vi "Test Get Audio Device Configuration.vi"(8 "error in (no error)":errorcluster) -> (0 "error out":errorcluster, 3 "Pass?":bool)   [LabVIEW 2020]
uses:
  G-Audio/Controls/Audio Device Config.ctl
  G-Audio/Controls/Audio Device Format.ctl
  G-Audio/Controls/Audio Device Advanced Config.ctl
  G-Audio/Private/Result To Error.vi
  G-Audio/Private/Audio Device Refnum To Value.vi
  <vilib>/Utility/error.llb/Error Cluster From Error Code.vi
  G-Audio/G-Audio.lvlib
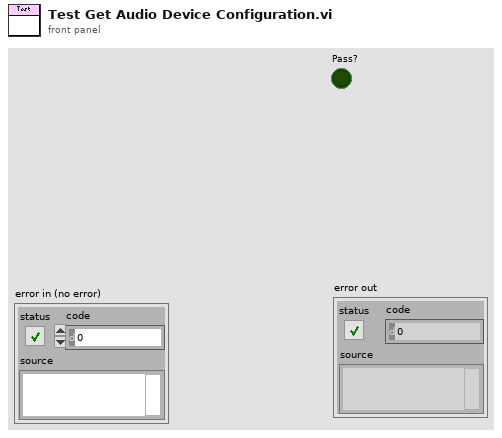
[diagram p1: front panel]
types:
  T1 = typedef "G-Audio.lvlib/Audio Device Advanced Config.ctl" = cluster{"Exclusive Mode":bool, "Period Size":u32, "Num Periods":u32}
  T2 = typedef "G-Audio.lvlib/Audio Device Config.ctl" = cluster{"Sample Rate (Hz)":u32, "Channels":u32, "Format":T3}
  T3 = typedef "G-Audio.lvlib/Audio Device Format.ctl" = enum16{"Native", "U8", "I16", "I32", "SGL"}
  T4 = typedef "G-Audio.lvlib/Audio Device Refnum.ctl" = refnum<file>
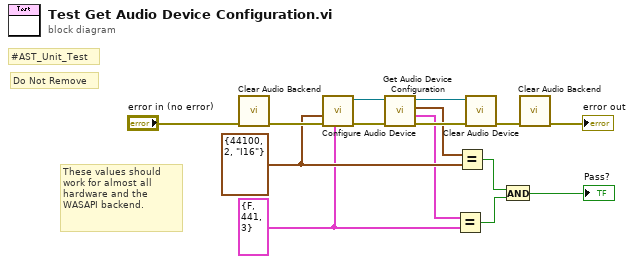
[diagram p0: block diagram]
diagram:
  w4 = T1 {"Exclusive Mode"=FALSE, "Period Size"=441, "Num Periods"=3} ("Advanced Config")
  w7 = T2 {"Sample Rate (Hz)"=44100, "Channels"=2, "Format"=enum."I16"} ("Device Config")
  # "These values should work for almost all hardware and the WASAPI backend."
  # "Do Not Remove"
  # "#AST_Unit_Test"
  n1 = call "Clear Audio Backend.vi"("error in (no error)"="error in (no error)") -> ("error out"=w14:errorcluster)  [unwired: 10 in]
  n2 = call "Configure Audio Device.vi"("Advanced Config"=w4, "error in (no error)"=w14, "Device Config"=w7) -> ("error out"=w11:errorcluster, "Audio Device Refnum"=w12:T4)  [unwired: 5 in, 2 out]
  n3 = call "Get Audio Device Configuration.vi"("error in (no error)"=w11, "Audio Device Refnum In"=w12) -> ("error out"=w10:errorcluster, "Audio Device Advanced Config"=w5:T1, "Audio Device Config"=w6:T2, "Audio Device Refnum Out"=w8:T4)  [unwired: 6 in]
  n4 = Equal?(x=w5, y=w4) -> (x = y?=w2:bool)
  n5 = Equal?(x=w6, y=w7) -> (x = y?=w3:bool)
  n6 = call "Clear Audio Device.vi"("error in (no error)"=w10, "Audio Device Refnum In"=w8) -> ("error out"=w9:errorcluster)  [unwired: 9 in]
  n7 = And(x=w3, y=w2) -> (x .and. y?=→"Pass?":bool)
  n8 = call "Clear Audio Backend.vi"("error in (no error)"=w9) -> ("error out"=→"error out":errorcluster)  [unwired: 10 in]
